vi "demo.vi"() -> ()   [LabVIEW 2019]
doc: "<License>This software is distributed under the BSD 3-Clause License. For the full license please see license.txt or visit www.labvolution.com/license</License>"
uses:
  SSH Library/Connection Info..cluster.ctl
  SSH Library/Password..cluster.ctl
  SSH Library/Private Public Key..cluster.ctl
  <vilib>/picture/3D Picture Control/Object/Create Object (name).vi
  SSH Library/connect_password.vi
  SSH Library/connect_key.vi
  SFTP Library/connect_password.vi
  SFTP Library/connect_key.vi
  <vilib>/Utility/file.llb/Read Delimited Spreadsheet (DBL).vi
  <vilib>/picture/3D Picture Control/Object/Add Object (no reference).vi
  SSH Library/LabSSH.lvlib
  SFTP Library/LabSFTP.lvlib
  <vilib>/picture/3D Picture Control/NI_3D Picture Control.lvlib
panel:
  out "诊断结果":bool
  out "诊断结论":string
  in  "选项卡控件":enum32{"实时监测", "参数设置", "文件传输"}(tab)
  in  "传感器选择":enum16{""}(ring)
  out "3D显示":refnum<vi>(3d-picture)
  in  "Sensor Values":dbl[](array[numeric])=[0.0, 0.0, 0.0, 0.0, 100.0] caption="传感器值"
  in  "Model File":path=path "C:/Users/1/Desktop/管道泄露检测系统/三维模型显示/hemisphere.STL" caption="模型文件"
  in  "Connection Info.":T1={"Remote"="192.168.1.106", "Username"="pi", "Port (22)"=22}
  in  "Password":T2={"Password"="zjl"}
  in  "Connection Type":enum16{"Password", "Private Key"}(ring)
  in  "Private_Public Key":T3
  in  "Expected Response":string="raspberrypi："
  out "isSshConnected":bool
  out "SSH Response":string="SSH connection closed\r\n"
  in  "file path (dialog if empty)":path=path "C:/Users/1/Desktop/管道泄露检测系统/download/datafile.dat" caption="Read file"
  in  "Remote File Path Up":string="/home/pi/leakad/"
  in  "Local File Up":path=path "C:/Users/1/Desktop/管道泄露检测系统/upload/txt.txt"
  in  "Remote File Path Down":string="/home/pi/leakad/datafile.dat"
  in  "Download Local File Path":path=path "C:/Users/1/Desktop/管道泄露检测系统/download"
  out "SFTP  Response":string="SFTP connection closed\r\n"
  out "isSftpConnected":bool
  in  "采集时间":i32=10
  out "次声波信号":dynamicdata(graph)
  in  "数据传输":bool
  in  "采集命令":string="cd /home/pi/leakad\nls\nsudo ./ADS1256 0 2000 5 1"
  in  "关闭":bool
  in  "连接设备":bool
  in  "error in (no error)":errorcluster
  out "Output":string="Linux raspberrypi 4.19.97-v7+ #1294 SMP Thu Jan 30 13:15:58 GMT 2020 armv7l\r\n\r\nThe programs included with the Debian GNU/Linux system are free software;\r\nthe exact distribution terms for each program are described in the\r\nindividual files in /usr/share/doc/*/copyright.\r\n\r\nDebian GNU/Linux comes with ABSOLUTELY NO WARRANTY, to the extent\r\npermitted by applicable law.\r\nLast login: Sun Apr 26 10:17:10 2020\r\r\npi@raspberrypi:~$ cd /home/pi/leakad\r\npi@raspberrypi:~/leakad$ ls\r\nADS1256  datafile.dat\r\npi@raspberrypi:~/leakad$ sudo ./ADS1256 0 2000 5 1\r\npi@raspberrypi:~/leakad$ "
  out "日期字符串":string="2020/4/26"
  out "时间字符串":string="10:47:37"
  # "管道泄漏监测系统"
  # "C:\\\\Working Folder\\\\ssh.git\\\\LabSSH\\\\raspberrypi_private_openssh.ppk"
  # "Upload File"
  # "Download File"
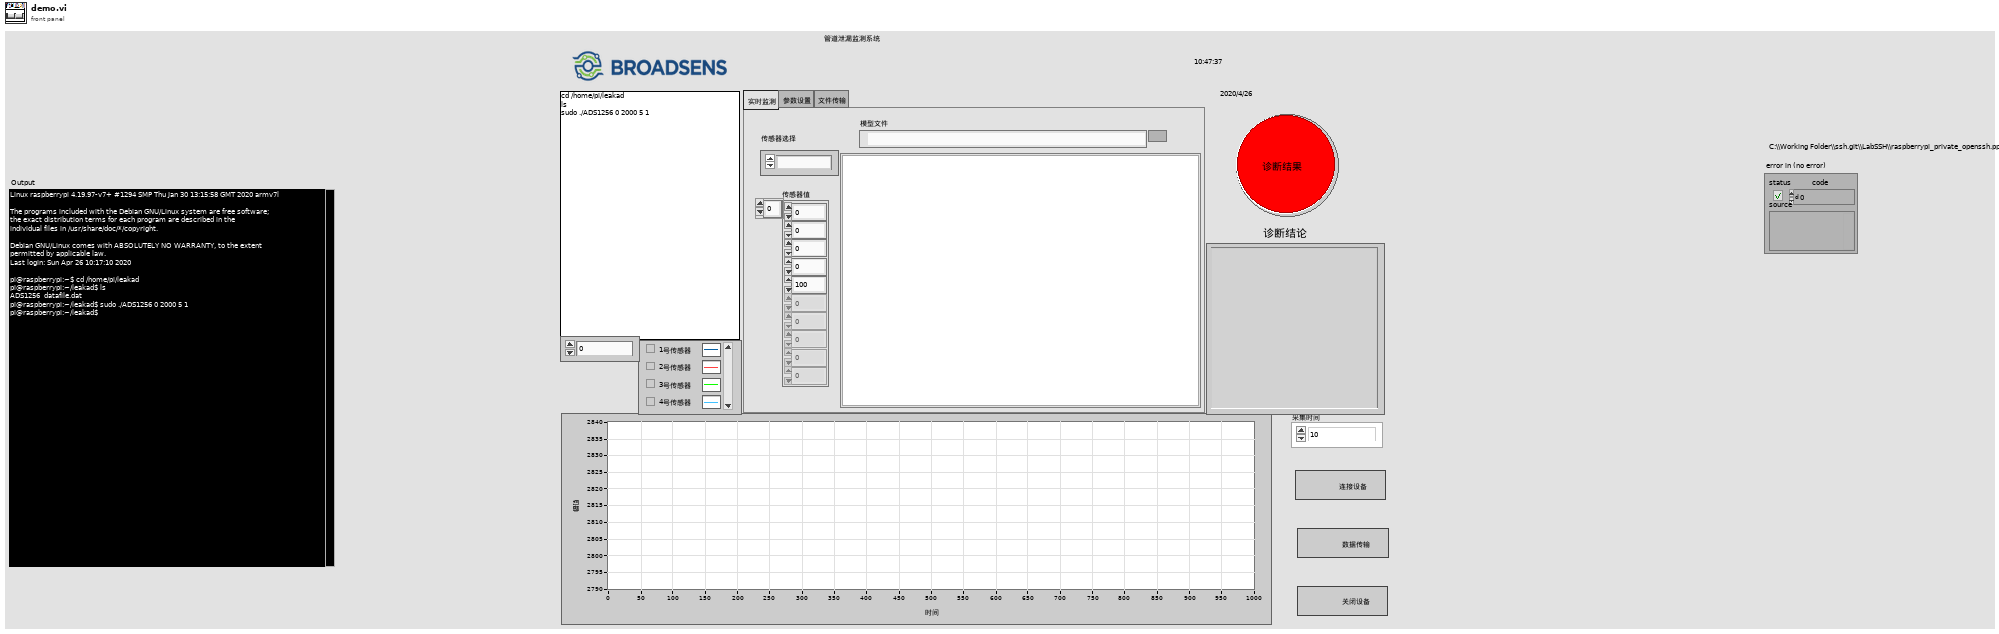
[diagram p1: front panel]
types:
  T1 = typedef "LabSSH.lvlib/Connection Info..cluster.ctl" = cluster{"Remote":string, "Username":string, "Port (22)":i32}
  T2 = typedef "LabSSH.lvlib/Password..cluster.ctl" = cluster{"Password":string}
  T3 = typedef "LabSSH.lvlib/Private Public Key..cluster.ctl" = cluster{"Private Key":path, "Passphrase":string}
  T4 = enum16{"None", "Spherical", "Flying", "Oriented"}
  T5 = enum32{"invalid app kind", "Development System", "Run Time System", "Student Edition", "Embedded LabVIEW", "Evaluation", "Custom"}
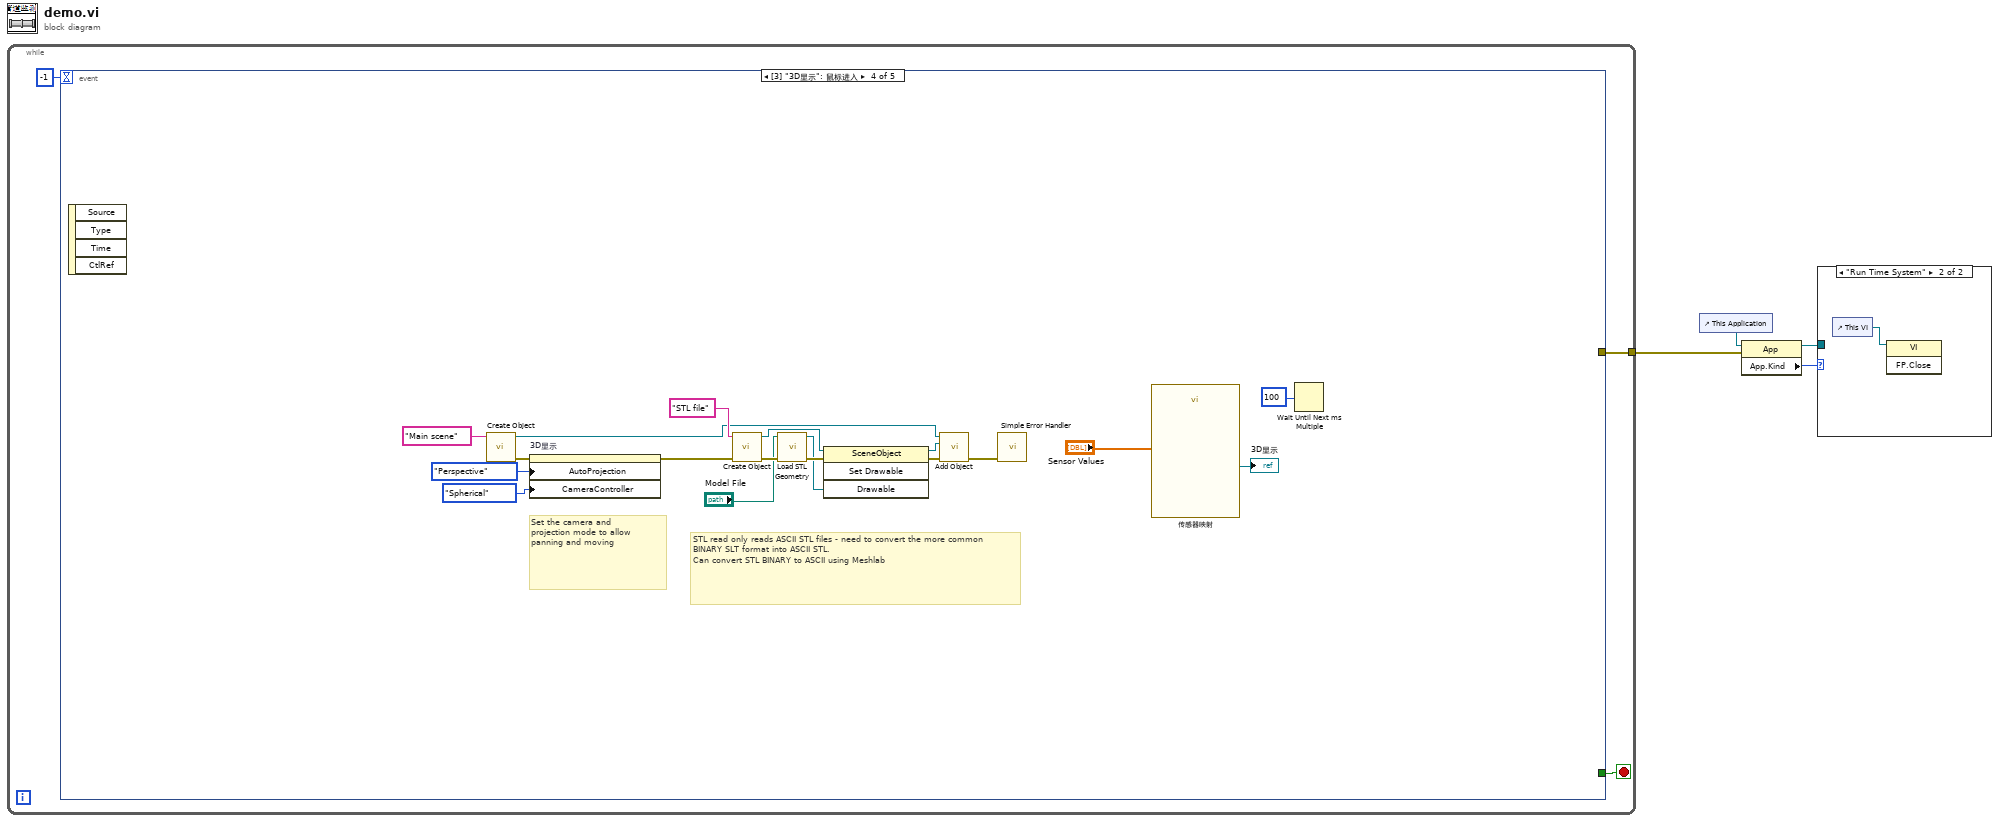
[diagram p0: block diagram]
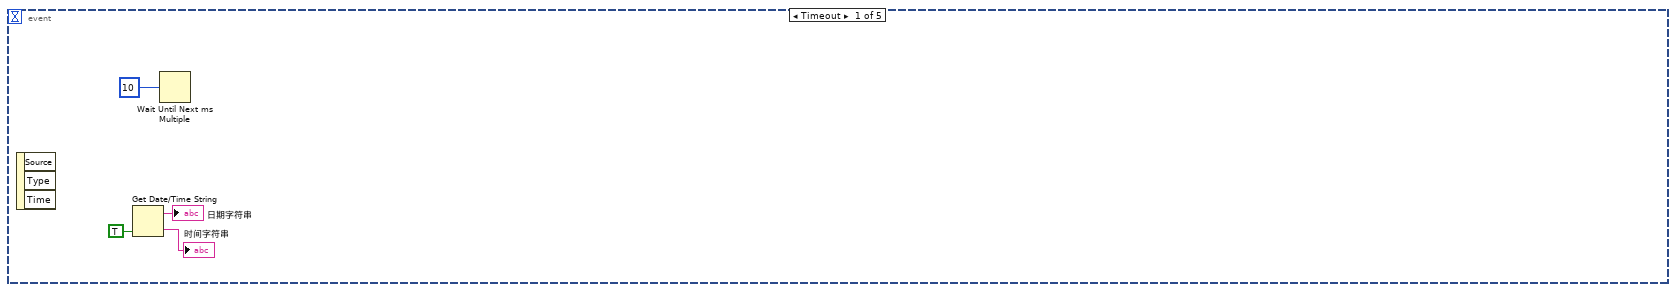
[diagram p2: hidden frame]
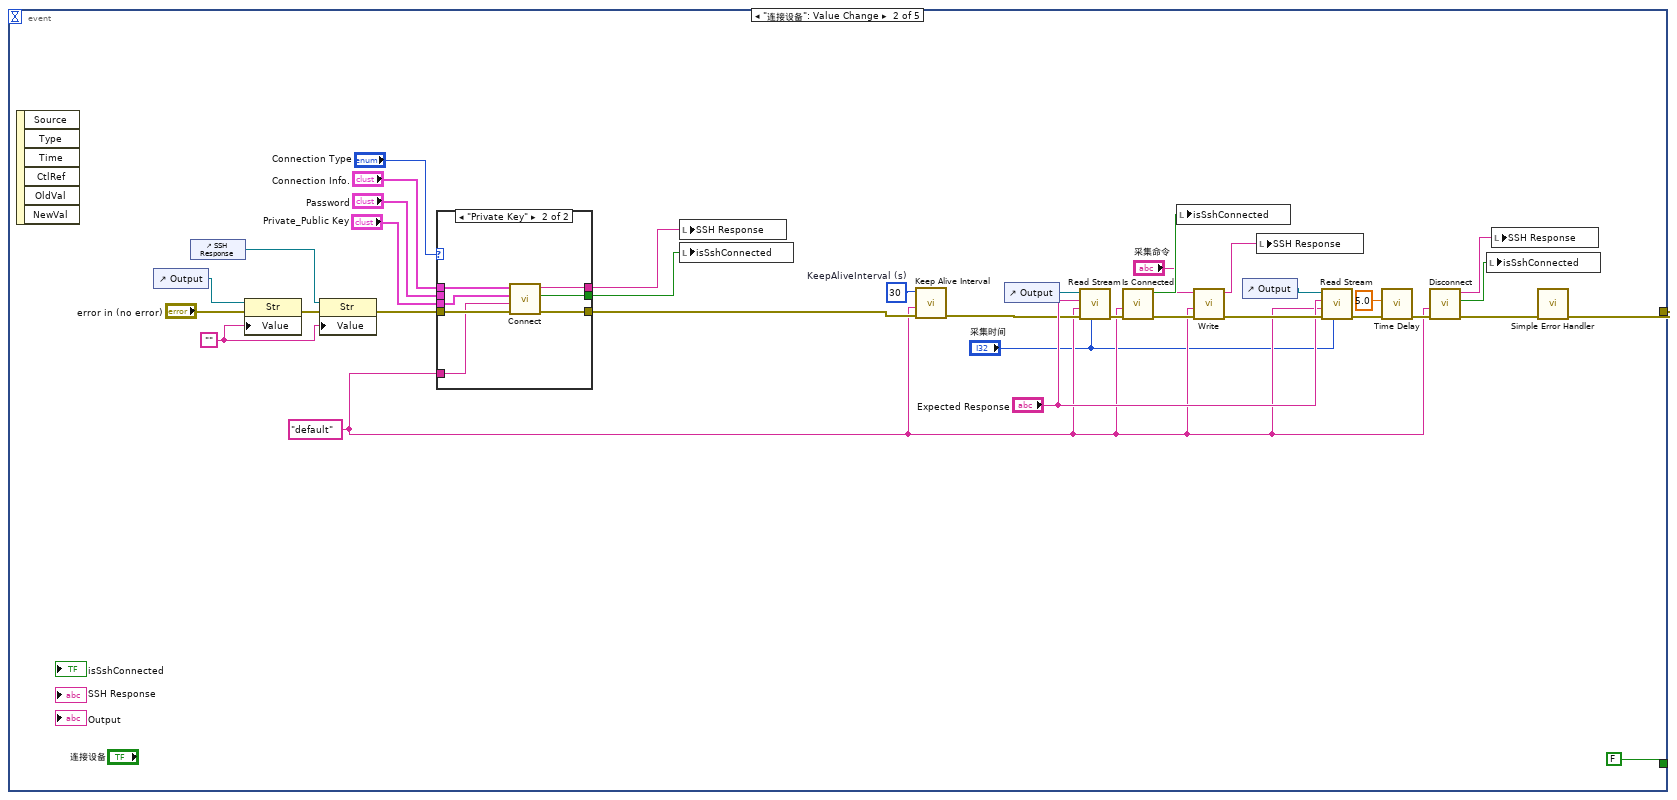
[diagram p3: hidden frame]
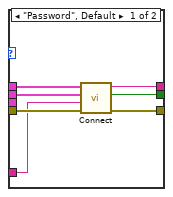
[diagram p4: hidden frame]
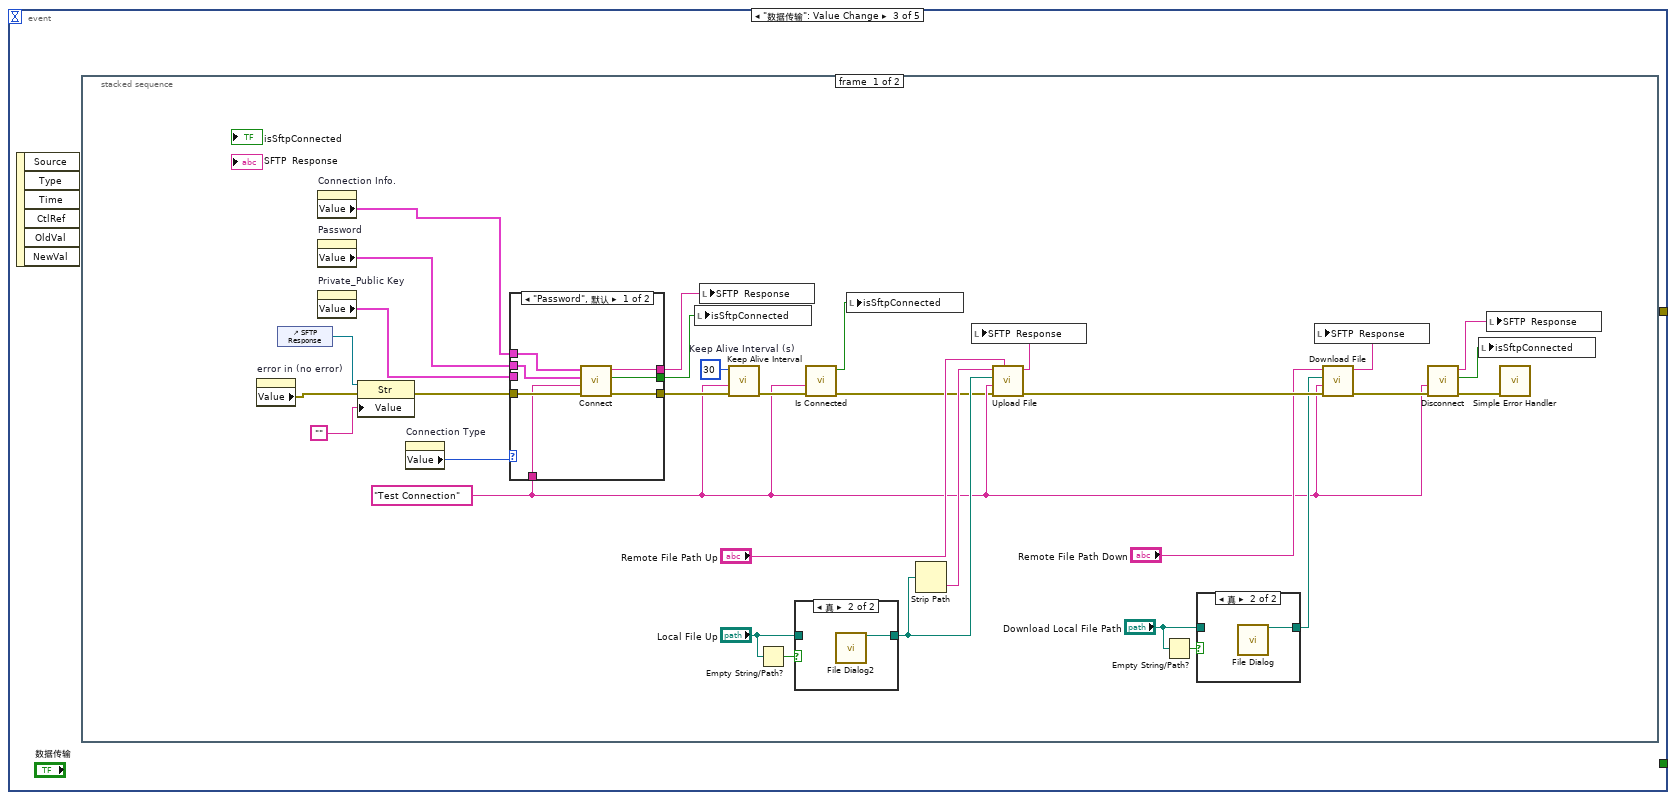
[diagram p5: hidden frame]
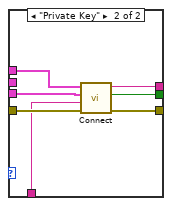
[diagram p7: hidden frame]
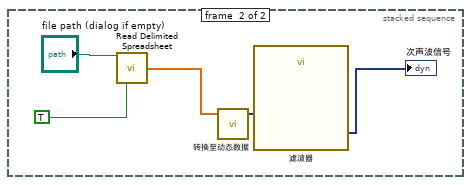
[diagram p9: hidden frame]
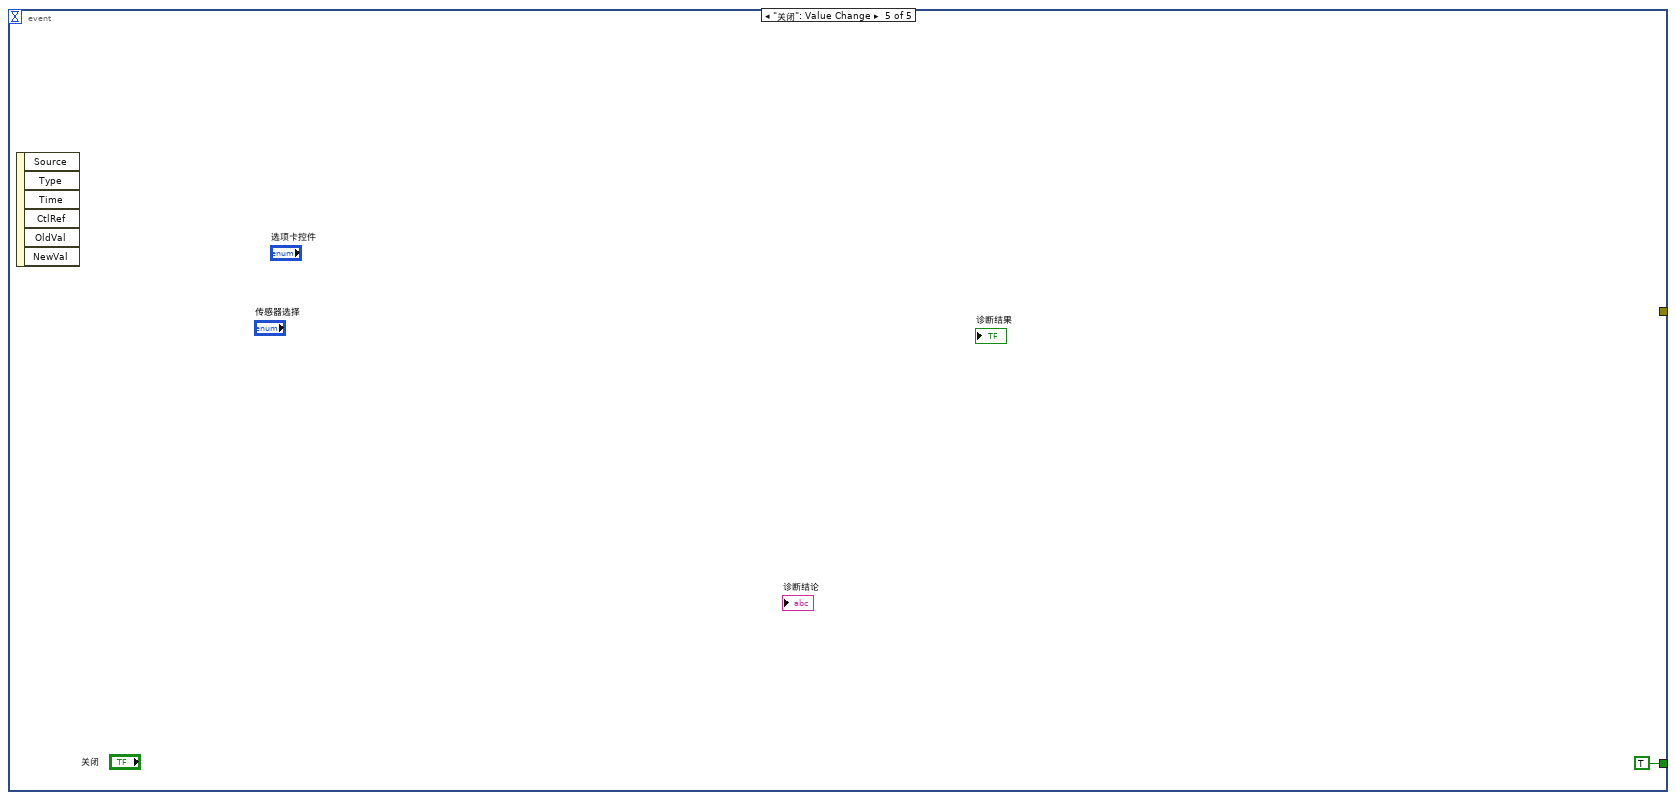
[diagram p10: hidden frame]
diagram:
  n1 = while {
    tunnel: [w6] -> w3
    stop <- w7 stop-if-true
    n2 = event shown="[3] \"3D显示\": 鼠标进入" {
      selector: _ -> [_ _ _ _ _]
      dyn-events: _ -> [_ _ _ _ _]
      timeout: -1 -> [_ _ _ _ _]
      tunnel: [_ FALSE _ _ TRUE] -> w7
      tunnel: [_ w20 _ _ _] -> w6
      event Timeout {
        n3 = event-data() -> ()  [unwired: 1 in, 3 out]
        n4 = Get Date/Time String(want seconds? (F)=TRUE ("需要秒？(F)")) -> (date string=→"日期字符串":string, time string=→"时间字符串":string)  [unwired: 2 in]
        n5 = Wait Until Next ms Multiple(millisecond multiple=u32 10 ("毫秒倍数")) -> ()  [unwired: 1 out]
      }
      event "连接设备": Value Change {
        w13 = "default" ("Connection Name")
        w17 = 30  # KeepAliveInterval (s)
        w28 = ""
        n6 = event-data() -> ()  [unwired: 1 in, 6 out]
        n7 = control-ref of="Output"() -> (w31:refnum<vi>)
        n8 = control-ref of="SSH Response"() -> (w29:refnum<vi>)
        n9 = property class="Str"(reference=w31, error in="error in (no error)", "Value"=w28) -> (error out=w32:errorcluster)  [unwired: 1 out]
        n10 = property class="Str"(reference=w29, error in=w32, "Value"=w28) -> (error out=w30:errorcluster)  [unwired: 1 out]
        n11 = case shown="\"Private Key\"" "Connection Type" {
          tunnel: [w52 w57] -> w18
          tunnel: "Connection Info." -> [w51 w59]
          tunnel: "Password" -> [w50 _]
          tunnel: [w49 w56] -> w40
          tunnel: [w48 w55] -> w35
          tunnel: w30 -> [w47 w58]
          tunnel: "Private_Public Key" -> [_ w54]
          tunnel: w13 -> [w46 w53]
          frame "Password", Default {
            n12 = call-poly "Connect.vi"("error in (no error)"=w47, "Connection Name"=w46, "Password"=w50, "Connection Info."=w51) -> ("error out"=w52:errorcluster, "isSshConnected"=w49:bool, "Return String"=w48:string)  [unwired: 5 in]
          }
          frame "Private Key" {
            n13 = call-poly "Connect.vi"("error in (no error)"=w58, "Connection Name"=w53, "Private_Public Key"=w54, "Connection Info."=w59) -> ("error out"=w57:errorcluster, "isSshConnected"=w56:bool, "Return String"=w55:string)  [unwired: 5 in]
          }
        }
        n14 = local write "SSH Response"(w35) -> ()
        n15 = local write "isSshConnected"(w40) -> ()
        n16 = call "Keep Alive Interval.vi"("error in (no error)"=w18, "Connection Name"=w13, "KeepAliveInterval (s)"=w17) -> ("error out"=w19:errorcluster)  [unwired: 8 in]
        n17 = control-ref of="Output"() -> (w45:refnum<vi>)
        n18 = call "Read Stream.vi"("Timout (s)"="采集时间", "error in (no error)"=w19, "Connection Name"=w13, "Expected Response"="Expected Response", "Output ref"=w45) -> ("error out"=w41:errorcluster)  [unwired: 6 in]
        n19 = call "Is Connected.vi"("error in (no error)"=w41, "Connection Name"=w13) -> ("error out"=w38:errorcluster, "isSshConnected"=w39:bool)  [unwired: 8 in]
        n20 = local write "isSshConnected"(w39) -> ()
        n21 = call "Write.vi"("error in (no error)"=w38, "Connection Name"=w13, "Command"="采集命令") -> ("error out"=w36:errorcluster, "Return String"=w34:string)  [unwired: 7 in]
        n22 = control-ref of="Output"() -> (w37:refnum<vi>)
        n23 = local write "SSH Response"(w34) -> ()
        n24 = call "Read Stream.vi"("Timout (s)"="采集时间", "error in (no error)"=w36, "Connection Name"=w13, "Expected Response"="Expected Response", "Output ref"=w37) -> ("error out"=w23:errorcluster)  [unwired: 6 in]
        n25 = call "Time Delay"("error in (no error)"=w23, "Delay Time (s)"=5.0) -> ("error out"=w22:errorcluster)  [unwired: 9 in]
        n26 = call "Disconnect.vi"("error in (no error)"=w22, "Connection Name"=w13) -> ("error out"=w33:errorcluster, "isSshConnected"=w15:bool, "Return String"=w16:string)  [unwired: 7 in]
        n27 = local write "isSshConnected"(w15) -> ()
        n28 = local write "SSH Response"(w16) -> ()
        n29 = call <vilib>:"Simple Error Handler.vi"("error in (no error)"=w33) -> ("error out"=w20:errorcluster)  [unwired: 4 in, 4 out]
      }
      event "数据传输": Value Change {
        n30 = event-data() -> ()  [unwired: 1 in, 6 out]
        n31 = stacked-sequence {
          frame #0 {
            w61 = "Test Connection" ("Connection Name")
            w74 = 30  # Keep Alive Interval (s)
            n32 = property on="error in (no error)" class="Clust (严格)"() -> ("Value"=w62:errorcluster)  [unwired: 2 in, 2 out]
            n33 = control-ref of="SFTP  Response"() -> (w84:refnum<vi>)
            n34 = property on="Connection Info." class="Clust (严格)"() -> ("Value"=w66:T1)  [unwired: 2 in, 2 out]
            n35 = property on="Password" class="Clust (严格)"() -> ("Value"=w63:T2)  [unwired: 2 in, 2 out]
            n36 = property on="Private_Public Key" class="Clust (严格)"() -> ("Value"=w65:T3)  [unwired: 2 in, 2 out]
            n37 = property class="Str"(reference=w84, error in=w62, "Value"="") -> (error out=w85:errorcluster)  [unwired: 1 out]
            n38 = property on="Connection Type" class="Enum (严格)"() -> ("Value"=w64:enum16{"Password", "Private Key"})  [unwired: 2 in, 2 out]
            n39 = case shown="\"Password\", 默认" w64 {
              tunnel: [w100 w106] -> w75
              tunnel: [w99 w105] -> w91
              tunnel: [w98 w104] -> w89
              tunnel: w85 -> [w97 w107]
              tunnel: w61 -> [w96 w103]
              tunnel: w66 -> [w95 w102]
              tunnel: w65 -> [_ w101]
              tunnel: w63 -> [w94 _]
              frame "Password", Default {
                n40 = call-poly "Connect.vi"("error in (no error)"=w97, "Connection Name"=w96, "Password"=w94, "Connection Info."=w95) -> ("error out"=w100:errorcluster, "isSftpConnected"=w99:bool, "Return String"=w98:string)  [unwired: 5 in]
              }
              frame "Private Key" {
                n41 = call-poly "Connect.vi"("error in (no error)"=w107, "Connection Name"=w103, "Private_Public Key"=w101, "Connection Info."=w102) -> ("error out"=w106:errorcluster, "isSshConnected"=w105:bool, "Return String"=w104:string)  [unwired: 5 in]
              }
            }
            n42 = local write "isSftpConnected"(w91) -> ()
            n43 = local write "SFTP  Response"(w89) -> ()
            n44 = call "Keep Alive Interval.vi"("error in (no error)"=w75, "Connection Name"=w61, "Keep Alive Interval (s)"=w74) -> ("error out"=w76:errorcluster)  [unwired: 8 in]
            n45 = Empty String/Path?(string/path="Local File Up") -> (empty?=w73:bool)
            n46 = case shown="真" w73 {
              tunnel: [w92 w93] -> w68
              tunnel: "Local File Up" -> [w92 _]
              frame False {
              }
              frame True {
                n47 = call "File Dialog2"() -> ("selected path"=w93:path)  [unwired: 12 in, 3 out]
              }
            }
            n48 = call "Is Connected.vi"("error in (no error)"=w76, "Connection Name"=w61) -> ("error out"=w60:errorcluster, "isSshConnected"=w90:bool)  [unwired: 8 in]
            n49 = local write "isSftpConnected"(w90) -> ()
            n50 = Strip Path(path=w68) -> (name=w78:string)  [unwired: 1 out]
            n51 = call "Upload File.vi"("Remote Folder Path"="Remote File Path Up", "error in (no error)"=w60, "Connection Name"=w61, "Local File Path"=w68, "Remote File Name"=w78) -> ("error out"=w81:errorcluster, "Return String"=w82:string)  [unwired: 5 in]
            n52 = local write "SFTP  Response"(w82) -> ()
            n53 = Empty String/Path?(string/path="Download Local File Path") -> (empty?=w71:bool)
            n54 = case shown="真" w71 {
              tunnel: [w108 w109] -> w69
              tunnel: "Download Local File Path" -> [w108 _]
              frame False {
              }
              frame True {
                n55 = call "File Dialog"() -> ("selected path"=w109:path)  [unwired: 12 in, 3 out]
              }
            }
            n56 = call "Download File.vi"("error in (no error)"=w81, "Connection Name"=w61, "Local File Path"=w69, "Remote File Path"="Remote File Path Down") -> ("error out"=w80:errorcluster, "Return String"=w79:string)  [unwired: 6 in]
            n57 = local write "SFTP  Response"(w79) -> ()
            n58 = call "Disconnect.vi"("error in (no error)"=w80, "Connection Name"=w61) -> ("error out"=w87:errorcluster, "isSshConnected"=w86:bool, "Return String"=w88:string)  [unwired: 7 in]
            n59 = local write "isSftpConnected"(w86) -> ()
            n60 = local write "SFTP  Response"(w88) -> ()
            n61 = call <vilib>:"Simple Error Handler.vi"("error in (no error)"=w87) -> ()  [unwired: 4 in, 5 out]
          }
          frame #1 {
            n62 = call-poly <vilib>:"Read Delimited Spreadsheet.vi"("file path (dialog if empty)"="file path (dialog if empty)", "transpose? (F)"=TRUE) -> ("first row"=w110:dbl[])  [unwired: 8 in, 5 out]
            n63 = call "转换至动态数据"("Array"=w110) -> ("Dynamic Data Type"=w112:dynamicdata)  [unwired: 3 in]
            n64 = call "滤波器"("Signal"=w112) -> ("Filtered Signal"=→"次声波信号":dynamicdata)  [unwired: 9 in, 1 out]
          }
        }
      }
      event "3D显示": Mouse Enter {
        # "Set the camera and projection mode to allow panning and moving"
        # "STL read only reads ASCII STL files - need to convert the more common BINARY SLT format into ASCII STL.\nCan convert STL BINARY to ASCII using Meshlab"
        n65 = event-data() -> ()  [unwired: 1 in, 4 out]
        n66 = call-poly <vilib>:"Create Object.vi"("Name"="Main scene") -> ("error out"=w121:errorcluster, "Scene:New Object"=w118:refnum<vi>)  [unwired: 9 in]
        n67 = property on="3D显示" class="SceneGraphDisp (严格)"(error in=w121, "AutoProjection"=enum16{"None", "Perspective", "Orthographic"}."Perspective" ("Automatic Projection Mode"), "CameraController"=T4."Spherical" ("Camera Controller:Type")) -> (error out=w119:errorcluster)  [unwired: 1 in, 1 out]
        n68 = call-poly <vilib>:"Create Object.vi"("error in (no error)"=w119, "Name"="STL file") -> ("error out"=w127:errorcluster, "Scene:New Object"=w128:refnum<vi>)  [unwired: 8 in]
        n69 = call <vilib>:"Load STL Geometry.vi"("error in (no error)"=w127, "Model File"="Model File") -> ("error out"=w132:errorcluster, "New Mesh Refnum"=w131:refnum<vi>)  [unwired: 8 in]
        n70 = invoke on="调用节点" class="SceneObject" method="Set Drawable"(reference=w128, error in=w132, "Drawable"=w131) -> (reference out=w126:refnum<vi>, error out=w125:errorcluster)  [unwired: 1 in, 2 out]
        n71 = call-poly <vilib>:"Add Object.vi"("error in (no error)"=w125, "New Object In"=w126, "Scene Object In"=w118) -> ("error out"=w124:errorcluster)  [unwired: 7 in, 1 out]
        n72 = call <vilib>:"Simple Error Handler.vi"("error in (no error)"=w124) -> ()  [unwired: 4 in, 5 out]
        n73 = call "传感器映射"("Sensor Values"="Sensor Values") -> ("Scene Ref Out"=→"3D显示":refnum<vi>)  [unwired: 9 in, 1 out]
        n74 = Wait Until Next ms Multiple(millisecond multiple=u32 100 ("毫秒倍数")) -> ()  [unwired: 1 out]
      }
      event "关闭": Value Change {
        n75 = event-data() -> ()  [unwired: 1 in, 6 out]
      }
    }
  }
  n76 = control-ref of="This Application"() -> (w4:refnum<vi>)
  n77 = property class="App"(reference=w4, error in=w3) -> (reference out=w1:refnum<vi>, "App.Kind"=w2:T5)  [unwired: 1 out]
  n78 = case shown="\"Run Time System\"" w2 {
    tunnel: w1 -> [_ _]
    frame "invalid app kind", Default {
    }
    frame "Run Time System" {
      n79 = control-ref of="This VI"() -> (w134:refnum<vi>)
      n80 = invoke class="VI" method="FP.Close"(reference=w134) -> ()  [unwired: 2 in, 3 out]
    }
  }
